vi "oopAPI_RX (SAP)_1.vi"() -> ()   [LabVIEW 2020]
uses:
  src/AIM664LV.lvlib
  <extravilib>/ChannelInstances/Tag-bool.lvlib
  <vilib>/platform/TimedLoop/XDataNode/XDataNode.xnode
  <vilib>/Platform/TimedLoop/XDataNode/nitl_modes.ctl
  <vilib>/Platform/TimedLoop/XDataNode/XDNodeRunTimeDep.lvlib
  <vilib>/Platform/TimedLoop/XDataNode/wakeup.ctl
  <vilib>/Platform/TimedLoop/XDataNode/timing_clust.ctl
  src/_polimorphicInstances/udpPort/Fdx Create Udp Port (RX-SAP).vi
  src/_polimorphicInstances/session/Fdx Create Session (Rx-VL-Oriented).vi
  src/_polimorphicInstances/control/Fdx Start (Rx).vi
  src/bsp/AFDX_Receive/Fdx Create Rx VL.vi
  src/_polimorphicInstances/session/Fdx Close Session (Port).vi
  src/_polimorphicInstances/control/Fdx Stop (Rx).vi
  src/_controls/comm_computedMAC-IP.ctl
  src/_controls/sap_config_rx.ctl
  src/_controls/comm_verification_rx.ctl
panel:
  out "MsgErrorCount":u32
  out "Duplicated":bool
  in  "VL Config":T1={"VlId"=0, "VLRange"=0, "VerificationMode"=0, "Bag"=0, "Jitter"=0, "MaxFrameLength"=0, "MaxSkew"=0, "VLBufSize"=32768, "FilterMode"=0, "FilterPosition"=0, "Padding"=0, "FilterMask"=0, "FilterData"=0, "MinFrameLength"=0} {"FilterMode" items=["FDX_RX_VL_FLT_DIS", "FDX_RX_VL_FLT_ENA ", "FDX_RX_VL_FLT_ENA_INV"]; "MaxFrameLength" format="%.0x"; "VerificationMode" items=["FDX_RX_VL_CHECK_ENA_DEFAULT"=65535, "FDX_RX_VL_CHECK_REDMAM"=16, "DX_RX_VL_CHECK_TRAFIC"=8, "FDX_RX_VL_CHECK_FRAMESIZE"=4, "FDX_RX_VL_CHECK_SNINTEG"=2, "FDX_RX_VL_CHECK_INVPAC"=1, "FDX_RX_VL_CHECK_DISA"=0]}
  in  "SapPort Config":T2
  out "FramesPerSecond":u32[](array[numeric])
  out "BytesPerSecond":u32[](array[numeric])
  out "src info":cluster{"ip src":u32, "udp src port":u32}
  in  "Processor":i32=-2
  in  "Period uS":i64=2000
  out "msg to read":u32
  in  "MsgCount(1)":u32=1
  in  "DefaultPayloadMode (Full)":u32(ring) items=["FDX_PAYLOAD_FULL", "FDX_PAYLOAD_IP_EXT", "FDX_PAYLOAD_IP", "FDX_PAYLOAD_MAC"]
  out "read time uS":u32(graph)
  out "BytesRead":u32
  out "irig time":T3
  in  "Port":u32=1
  in  "Board":u32
  out "current time":timestamp
  out "current irig time":T4={"SignOut"=-1509901600, "DayOut"=16, "HourOut"=8, "MinOut"=7, "SecondOut"=53, "MilliSecOut"=368, "MicroSecOut"=508, "NanoSecOut"=600, "InfoOut"=0, "Mode"=3}
  out "computedAddresses":T5 {"MACsrc" format="%.0x"}
  out "Data":u8[](array[numeric])=[1, 2, 3, 4, 0, 0, 0, 0, 0, 0, 0, 0, 0, 0, 0, 0, 0, 0, 0, 0, 0, 0, 0, 0, 0, 0, 0, 0, 0, 0, 0, 0, 0, 0, 0, 0, 0, 0, 0, 0, 0, 0, 0, 0, 0, 0, 0, 0, 0, 0, 0, 0, 0, 0, 0, 0, 0, 0, 0, 0, 0, 0, 0, 0, 0, 0, 0, 0, 0, 0, 0, 0, 0, 0, 0, 0, 0, 0, 0, 0, 0, 0, 0, 0, 0, 0, 0, 0, 0, 0, 0, 0, 0, 0, 0, 0, 0, 0, 0, 0] format="%.0x"
  in  "stop":bool
  out "PortInitOut":T6={"PortConfig"=0, "PortUsed"=1, "GlobalMemFree"=0, "SharedMemFree"=0} {"PortConfig" items=["FDX_SINGLE", "FDX_REDUNDANT"]}
  out "error out":errorcluster
  # "ARINC 664 - Receiving Service Access Point (SAP) Level 1"
  # "Overview: Setup the board to transmit package as raw frames.\nRequirement: One AIM ARINC-664 board with installed AIM ARINC 664 BSP.\nRestrictions: None.\nInstruction:\n1. Select the Board ID (0 if you have only one board in your system) and the port number. If you want to validate between two ports in one device, you can use tx board and Rx Board\n2. Run the VI.\n3. See the result in Current IRIG Time"
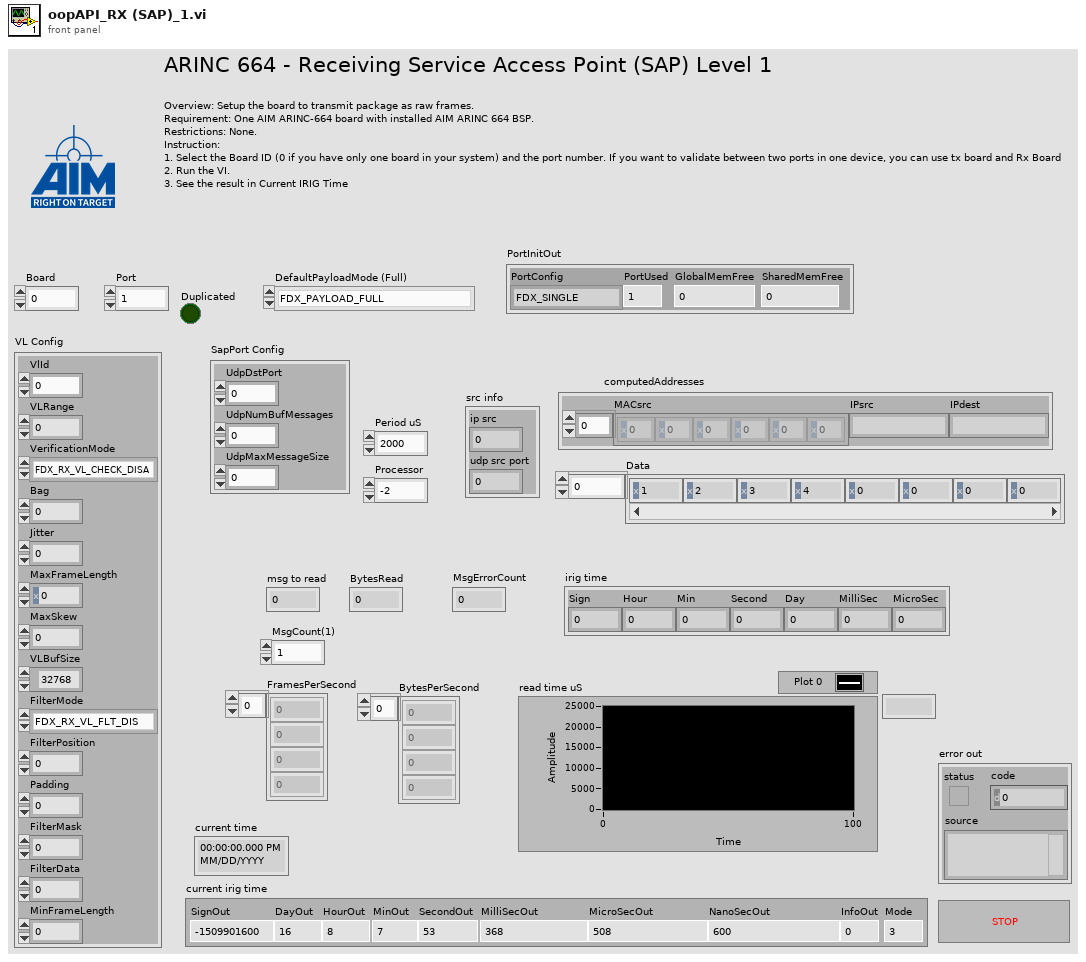
[diagram p1: front panel]
types:
  T1 = typedef "AIM664LV.lvlib/comm_verification_rx.ctl" = cluster{"VlId":u16, "VLRange":u32, "VerificationMode":u32, "Bag":u32, "Jitter":u32, "MaxFrameLength":u32, "MaxSkew":u32, "VLBufSize":u32, "FilterMode":u32, "FilterPosition":u32, "Padding":u32, "FilterMask":u32, "FilterData":u32, "MinFrameLength":u32}
  T2 = typedef "AIM664LV.lvlib/sap_config_rx.ctl" = cluster{"UdpDstPort":u16, "UdpNumBufMessages":u32, "UdpMaxMessageSize":u32}
  T3 = cluster{"Sign":i32, "Hour":u32, "Min":u32, "Second":u32, "Day":u32, "MilliSec":u32, "MicroSec":u32}
  T4 = cluster{"SignOut":i32, "DayOut":u32, "HourOut":u32, "MinOut":u32, "SecondOut":u32, "MilliSecOut":u32, "MicroSecOut":u32, "NanoSecOut":u32, "InfoOut":u32, "Mode":u32}
  T5 = typedef "AIM664LV.lvlib/comm_computedMAC-IP.ctl" = cluster{"MACsrc":u8[], "IPsrc":string, "IPdest":string}
  T6 = cluster{"PortConfig":u32, "PortUsed":u32, "GlobalMemFree":u32, "SharedMemFree":u32}
  T7 = typedef "XDNodeRunTimeDep.lvlib/timing_clust.ctl" = cluster{"Expected End [f-1]":u64, "Actual End [f-1]":u64, "Finished Late? [f-1]":bool, "Expected End [i-1]":u64, "Actual End [i-1]":u64, "Finished Late? [i-1]":bool, "Expected Start [i]":u64, "Actual Start [i]":u64, "Expected Start [f]":u64, "Actual Start [f]":u64, "Source Name":string, "Structure Name":string, "Period":i64, "Deadline":i64, "Offset":i64, "Start":i64, "Priority":i32, "Timeout":i32, "Mode":T8, "Wakeup Reason":T9, "Error":errorcluster, "Source Type":string, "Secondary Source Type":string, "Global End Time":u64, "Global Start Time":u64, "Frame Duration":u64, "Iteration Duration":u64, "Assigned CPU":i32, "I/O Scan Engine Mode":u32}
  T8 = typedef "XDNodeRunTimeDep.lvlib/nitl_modes.ctl" = enum32{"No Change", "Process missed periods, maintain original phase", "Discard missed periods, maintain original phase", "Process missed periods, ignore original phase", "Discard missed periods, ignore original phase"}
  T9 = typedef "XDNodeRunTimeDep.lvlib/wakeup.ctl" = enum32{"Normal", "Aborted", "Asynchronous wakeup", "Timing source error", "Timed loop error", "Timeout"}
  T10 = cluster{"TotalByteCount":u32[], "FrameGoodCount":u32[], "FrameErrorCount":u32[], "BytesPerSecond":u32[], "FramesPerSecond":u32[], "PhysErrorCount":u32[], "PreamErrorCount":u32[], "UnaligErrorCount":u32[], "CRCErrorCount":u32[], "IFGErrorCount":u32[], "IPErrorCount":u32[], "MACErrorCount":u32[], "NoSfdErrorCount":u32[], "VLLenErrorCount":u32[], "SNIntegrityErrorCount":u32[], "TrafShapingViolationCount":u32[], "MAC1Short":u32[], "MAC64To127Count":u32[], "MAC128To255Count":u32[], "MAC256To511Count":u32[], "MAC512To1023Count":u32[], "MAC1024To1518Count":u32[], "MACLong":u32[]}
  T11 = typedef "Tag-bool.lvlib/))Channel.ctl" = refnum<queue>
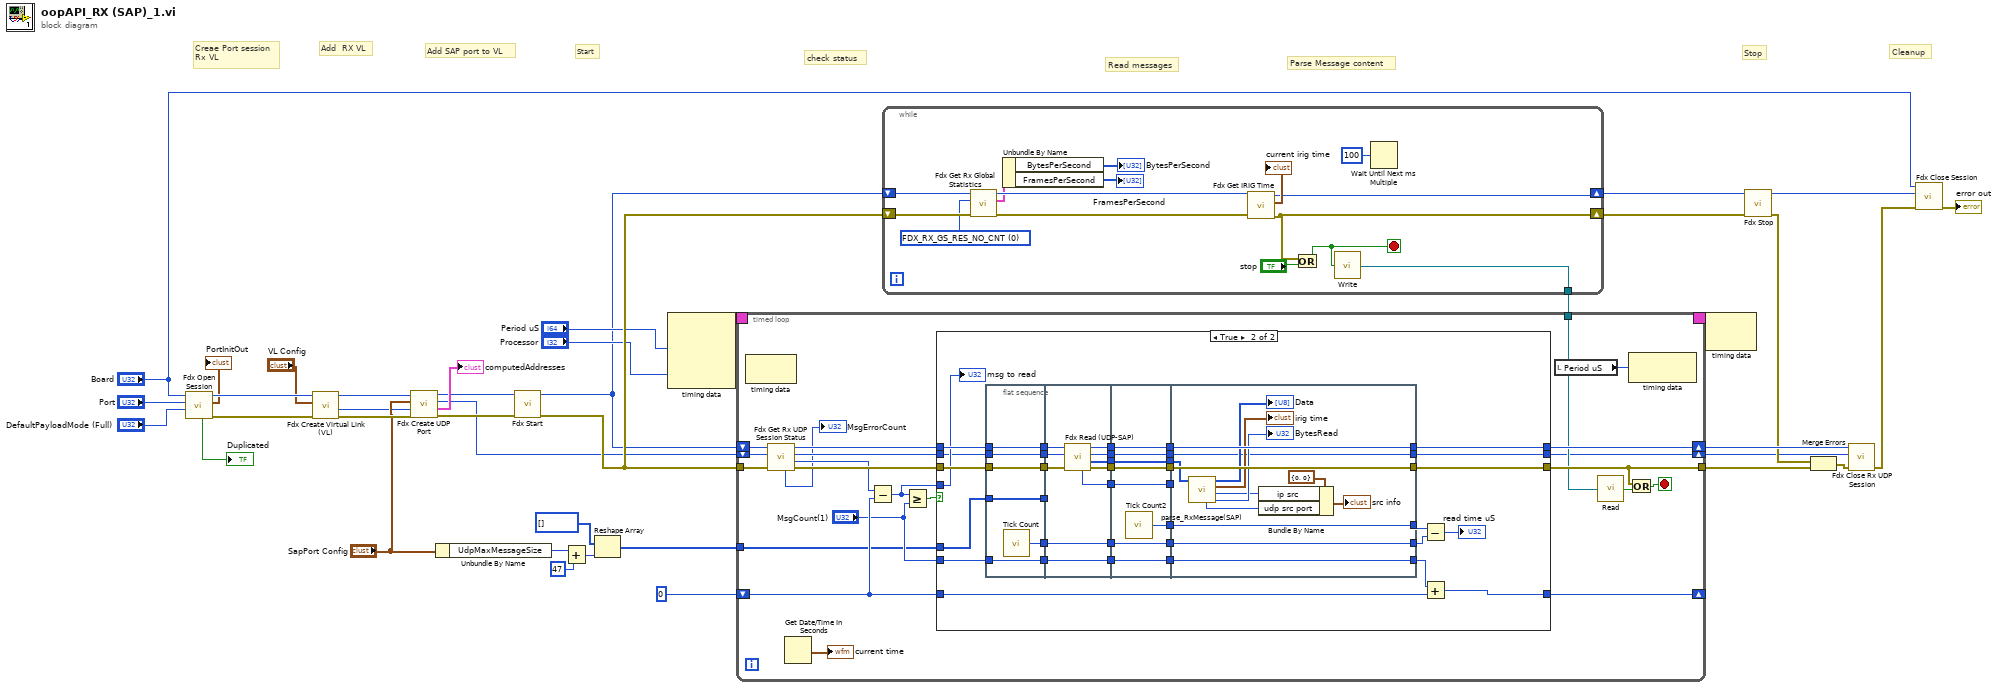
[diagram p0: block diagram]
diagram:
  # "Parse Message content"
  # "Cleanup"
  # "Stop"
  # "Read messages"
  # "check status"
  # "Start"
  # "Add SAP port to VL"
  # "Add  RX VL"
  # "Creae Port session\nRx VL"
  n1 = call-poly "Fdx Open Session.vi"("DefaultPayloadMode (Full)"="DefaultPayloadMode (Full)", "port"="Port", "board"="Board") -> ("error out"=w11:errorcluster, "PortInitOut"=→"PortInitOut":T6, "InstrumentHandle_port out"=w34:u32, "Duplicated"=→"Duplicated":bool)  [unwired: 3 in, 2 out]
  n2 = call-poly "Fdx Create Virtual Link (VL).vi"("error in (no error)"=w11, "VL Config"="VL Config", "InstrumentHandle_port in"=w34) -> ("error out"=w12:errorcluster, "VlId"=w6:u16, "InstrumentHandle_port out"=w13:u32)  [unwired: 6 in]
  n3 = call-poly "Fdx Create UDP Port.vi"("error in (no error)"=w12, "VlId"=w6, "SapPort Config"="SapPort Config", "port handle in"=w13) -> ("error out"=w38:errorcluster, "computedAddresses"=→"computedAddresses":T5, "sapPort handle out"=w4:u32, "port handle out"=w36:u32)  [unwired: 4 in]
  n4 = Unbundle By Name("SapPort Config") -> ("UdpMaxMessageSize"=w9:u32)
  n5 = call-poly "Fdx Start.vi"("error in (no error)"=w38, "InstrumentHandle_port in"=w36) -> ("error out"=w30:errorcluster, "InstrumentHandle_port out"=w5:u32)  [unwired: 8 in]
  n6 = Add(x=w9, y=u32 47) -> (x+y=w16:u32)
  n7 = Reshape Array(u8[] [] ("Buffer In"), w16) -> (w14:u8[])
  n8 = node-c288("Period uS", "Processor") -> (w21:T7)  [unwired: 2 in]
  n9 = while {
    tunnel: [w48] -> w26
    shift-right: [w51] -> w29
    shift-left: w5 -> [w53]
    shift-right: [w50] -> w28
    shift-left: w30 -> [w45]
    stop <- w49 stop-if-true
    w40 = u32 0 items=["FDX_RX_GS_RES_NO_CNT", "FDX_RX_GS_RES_ALL_CNT", "FDX_RX_GS_RES_ERR_CNT"] ("Control")
    n10 = call "Fdx Get Rx Global Statistics.vi"("error in (no error)"=w45, "Control"=w40, "InstrumentHandle_port in"=w53) -> ("error out"=w44:errorcluster, "GlobalStat Out"=w43:T10, "InstrumentHandle_port out"=w46:u32)  [unwired: 6 in]
    n11 = Unbundle By Name(w43) -> ("BytesPerSecond"=→"BytesPerSecond":u32[], "FramesPerSecond"=→"FramesPerSecond":u32[])
    n12 = call "Fdx Get IRIG Time.vi"("error in (no error)"=w44, "InstrumentHandle_board in"=w46) -> ("error out"=w50:errorcluster, "Curent Irig Time"=→"current irig time":T4, "InstrumentHandle_board out"=w51:u32)  [unwired: 7 in]
    n13 = Or(x=w50, y="stop") -> (x .or. y?=w49:bool)
    n14 = call <extravilib>:"Write.vi"("element"=w49) -> ("channel"=w48:T11)  [unwired: 1 out]
    n15 = Wait Until Next ms Multiple(millisecond multiple=u32 100) -> ()  [unwired: 1 out]
  }
  n16 = timed-loop {
    tunnel: w30 -> [w70]
    tunnel: [w73] -> w23
    tunnel: w26 -> [w71]
    shift-right: [w64] -> _
    shift-left: 0 -> [w66]
    timing: w21 -> [_]
    timing-out: [_] -> w20
    tunnel: w14 -> [w61]
    shift-right: [w55] -> w1
    shift-left: w4 -> [w60]
    shift-right: [w74] -> w31
    shift-left: w5 -> [w59]
    stop <- w76 stop-if-true
    n17 = node-c288() -> ()  [unwired: 1 in, 1 out]
    n18 = call "Fdx Get Rx UDP Session Status.vi"("error in (no error)"=w70, "UdpHandle in"=w60, "InstrumentHandle_port in"=w59) -> ("error out"=w68:errorcluster, "MsgCount"=w57:u32, "UdpHandle out"=w58:u32, "InstrumentHandle_port out"=w69:u32, "MsgErrorCount"=→"MsgErrorCount":u32)  [unwired: 4 in]
    n19 = Get Date/Time In Seconds() -> (seconds since 1Jan1904=→"current time":timestamp)
    n20 = Subtract(x=w57, y=w66) -> (x-y=w63:u32)
    n21 = Greater Or Equal?(x=w63, y="MsgCount(1)") -> (x >= y?=w67:bool)
    n22 = case shown="True" w67 {
      tunnel: w68 -> [w83 w106]
      tunnel: w69 -> [w84 w105]
      tunnel: [w84 w101] -> w74
      tunnel: [w83 w100] -> w73
      tunnel: "MsgCount(1)" -> [_ w90]
      tunnel: w66 -> [w82 w96]
      tunnel: [w82 w95] -> w64
      tunnel: w63 -> [_ w94]
      tunnel: w61 -> [_ w92]
      tunnel: w58 -> [w81 w88]
      tunnel: [w81 w85] -> w55
      frame False {
      }
      frame True {
        n23 = flat-sequence {
          tunnel: w106 -> [w125]
          tunnel: w105 -> [w126]
          tunnel: [w126] -> w120
          tunnel: [w125] -> w119
          tunnel: [w124] -> w118
          tunnel: [w123] -> w93
          tunnel: w92 -> [w123]
          tunnel: [w122] -> w91
          tunnel: w90 -> [w122]
          tunnel: [w121] -> w89
          tunnel: w88 -> [w121]
          tunnel: w120 -> [w131]
          tunnel: w119 -> [w132]
          tunnel: w118 -> [w136]
          tunnel: [w136] -> w117
          tunnel: [w135] -> w116
          tunnel: [w134] -> w115
          tunnel: [w133] -> w114
          tunnel: [w130] -> w113
          tunnel: [w129] -> w98
          tunnel: w93 -> [_]
          tunnel: w91 -> [w129]
          tunnel: w89 -> [w128]
          tunnel: [w127] -> w87
          tunnel: w117 -> [w144]
          tunnel: [w144] -> w112
          tunnel: [w143] -> w111
          tunnel: [w142] -> w110
          tunnel: w116 -> [w142]
          tunnel: [w141] -> w109
          tunnel: w115 -> [w141]
          tunnel: [w140] -> w108
          tunnel: w114 -> [w140]
          tunnel: [w139] -> w107
          tunnel: w113 -> [w139]
          tunnel: [w138] -> w99
          tunnel: w98 -> [w138]
          tunnel: w87 -> [w137]
          tunnel: [w137] -> w86
          tunnel: w112 -> [w158]
          tunnel: w111 -> [w157]
          tunnel: w110 -> [w156]
          tunnel: w109 -> [w155]
          tunnel: w108 -> [w153]
          tunnel: w107 -> [_]
          tunnel: w99 -> [w154]
          tunnel: w86 -> [w145]
          tunnel: [w158] -> w104
          tunnel: [w157] -> w102
          tunnel: [w156] -> w101
          tunnel: [w155] -> w100
          tunnel: [w154] -> w97
          tunnel: [w145] -> w85
          frame #0 {
            n24 = call "Tick Count"() -> ("Tick Count(uSec)"=w124:u32)
          }
          frame #1 {
            n25 = call "Fdx Read (UDP-SAP).vi"("error in"=w132, "UdpHandle in"=w128, "InstrumentHandle_port in"=w131) -> ("error out"=w134:errorcluster, "Data"=w133:u8[], "UdpHandle out"=w127:u32, "InstrumentHandle_port out"=w135:u32, "MsgRead"=w130:u32)  [unwired: 4 in]
          }
          frame #2 {
            n26 = call "Tick Count2"() -> ("Tick Count(uSec)"=w143:u32)
          }
          frame #3 {
            n27 = call "parse_RxMessage(SAP).vi"("ReadBuffer In"=w153) -> ("msg size"=→"BytesRead":u32, "ip src"=w146:u32, "IrigTime"=→"irig time":T3, "Message Data"=→"Data":u8[], "udp src port"=w147:u32)  [unwired: 6 in]
            n28 = Bundle By Name(cluster=cluster{"ip src":u32, "udp src port":u32} {"ip src"=0, "udp src port"=0} ("src info"), "ip src"=w146, "udp src port"=w147) -> (→"src info":cluster{"ip src":u32, "udp src port":u32})
          }
        }
        n29 = Subtract(x=w102, y=w104) -> (x-y=→"read time uS":u32)
        n30 = Add(x=w97, y=w96) -> (x+y=w95:u32)
        "msg to read" <- w94
      }
    }
    n31 = local read "Period uS"() -> (w62:i64)
    n32 = call <extravilib>:"Read.vi"("channel"=w71) -> ("element"=w72:bool)  [unwired: 1 in, 1 out]
    n33 = node-c288(w62) -> ()  [unwired: 1 out]
    n34 = Or(x=w73, y=w72) -> (x .or. y?=w76:bool)
  }
  n35 = node-c288(w20) -> ()  [unwired: 1 out]
  n36 = call-poly "Fdx Stop.vi"("error in (no error)"=w28, "InstrumentHandle_port in"=w29) -> ("error out"=w24:errorcluster, "InstrumentHandle_port out"=w2:u32)  [unwired: 8 in]
  n37 = Merge Errors(w24, w23) -> (w25:errorcluster)
  n38 = call "Fdx Close Rx UDP Session.vi"("error in (no error)"=w25, "UdpHandle in"=w1, "InstrumentHandle_port in"=w31) -> ("error out"=w27:errorcluster)  [unwired: 7 in, 1 out]
  n39 = call-poly "Fdx Close Session.vi"("error in (no error)"=w27, "InstrumentHandle_port in"=w2, "InstrumentHandle_board in"="Board") -> ("error out"=→"error out":errorcluster)  [unwired: 8 in]
